vi "PC Streaming Host with slow.vi"() -> ()   [LabVIEW 2012]
uses:
  <vilib>/userdefined/High Color/nirio_resource_hc.ctl
  <vilib>/FPGAPlugInAG/PXI-7951R/niLvFpga_Open_PXI-7951R.vi
  <vilib>/rvi/interface/common/dynamic/niFpgaDynamicAddResources.vi
  <vilib>/Utility/error.llb/Error Cluster From Error Code.vi
  <vilib>/rvi/errors/niLvFpgaAdjustHostInterfaceError.vi
  <vilib>/FPGAPlugInAG/Dynamic/niLvFpga_Close_Dynamic.vi
  <vilib>/rvi/interface/nirviOpenFPGA/nirviOpenFPGA.xnode
  FPGA Bitfiles/ModuDAQ_FPGATarget_TopLevelFPGAw8ra_+uETqx0Rcow.lvbitx
  <vilib>/rvi/interface/nirviReadWriteControl/nirviReadWriteControl.xnode
  <vilib>/rvi/interface/nirviMethod/nirviMethod.xnode
  <vilib>/rvi/interface/nirviCloseFPGA/nirviCloseFPGA.xnode
  <vilib>/ptbypt/NI_PtbyPt.lvlib
  <vilib>/rvi/interface/Simulation/niFpgaSimulationCallBeginRW.vi
  RT_binary.vi
  NiFpgaLv.dll
  <vilib>/FPGAPlugInAG/Dynamic/niLvFpga_ReadFifo_Dynamic.vi
  <vilib>/rvi/errors/niLvFpgaMergeErrorWithErrorCode.vi
panel:
  out "created path":path
  out "File name":string
  out "Total Data Chunks to Write":dbl
  in  "Tab Control":T1(tab)
  in  "Write mode":bool
  out "directory exists - please wait":u8(slide)
  out "directory ok":bool
  in  "Write Enable":bool
  in  "File Path":path=path "D:/Users/reuterc/Desktop"
  out "File Writing Progress (%)":dbl(slide) scale=0.0..100.0
  in  "Slow Control On":bool
  in  "Fast Data On":bool
  in  "Number of Files to Write":u32=1
  in  "IP Address of NIST Time Server":string(combo)
  in  "VISA resource name":refnum<visa-resource-name>="COM5"
  in  "General Cluster":cluster{"Location":i16} {"Location" items=["Purdue", "NIKHEF", "Zurich", "???"]}
  in  "PXI address":T2 caption="RIO Device"
  in  "Channel Cluster":T3={"det_type"=[], "voltage"=[], "Serial numbers"=[], "Sources"=[], "Trigger level"=[4000, 4000, 4000, 4000, 4000, 4000, 4000, 4000], "Channel On/Off"=[], "Number of Channels"=8}
  in  "Testpulse Cluster":T4={"Master Pulser On/Off"=FALSE, "Testpulse Turnaround Time (samples)"=14, "Pulse Separation (samples)"=0, "Pulse duration (samples)"=0}
  out "Samples per Data Chunk":u32
  in  "DAQ Info Cluster":T5={"Data Chunks per File"=1000, "Samples per Waveform"=95, "Pretrigger Samples"=15, "circular buffer length (samples)"=1000, "Waveforms per Data Chunk"=5000} {"Waveforms per Data Chunk" format="%.2p"}
  out "Average Throughput":dbl(graph)
  out "Loop Time":u32
  out "Inst. Throughput":dbl format="%#_6p"
  out "Elements in FIFO":u32(graph)
  out "FIFO Overflow":bool
  out "Current Chunk":u32
  out "Current File":i32
  out "Waveform Graph":dynamicdata(graph)
  out "Channel number displayed":i16=-1
  in  "Arduino read rate (Hz)":dbl=1.0
  out "read buffer":string
  out "array 2":string[](array[string])
  out "Arduino read failed":bool
  out "Slow time":u64
  out "data":dbl[](array[numeric])
  in  "XON Character":u8=17 format="%.0x"
  in  "XOFF Character":u8=19 format="%.0x"
  out "Slow Cluster":T6={"Number of Slow Parameters"=0, "UTC format?"=TRUE, "Sensor Upper bounds"=[85, 1000000, 8000, 8000, 8000, 14000, 99, 33000], "Sensor Lower bounds"=[-40, 0, -8000, -8000, -8000, -14000, 0, -33000], "datanames"=[], "Descriptions"=[]}
  out "FPGA Timestamp (s)":u64
  out "Temperature":dbl(graph)
  out "Pressure":dbl(graph)
  out "magnetic field y coordinate":dbl(graph)
  out "total magnetic field":dbl(graph)
  out "magnetic field z coordinate":dbl(graph)
  out "magnetic field x coordinate":dbl(graph)
  out "humidity":dbl(graph)
  out "XML String":string
  out "Slow XML":string
  out "error out":errorcluster
  out "NIST Time":u64
  out "NIST Time Failed to Read":bool
  in  "Minutes to wait":u32=5 min=3
  out "UTC format":bool=TRUE
  out "Stopped":bool
  in  "stop 2":bool
  in  "stop":bool
  # "Write continuously"
  # "Write finite number of files"
  # "Program will stop when number of Files to Write is Complete OR if stop is pressed."
  # "TODO: Make this look like the \"detectors\" tab"
  # "Waveform/Data Chunk information"
  # "To compare directly on a scope: Horizontal scale: 200 ns/div Vertical scale: ~100 mV/div If 15 pretriggers, delay = 700 ns"
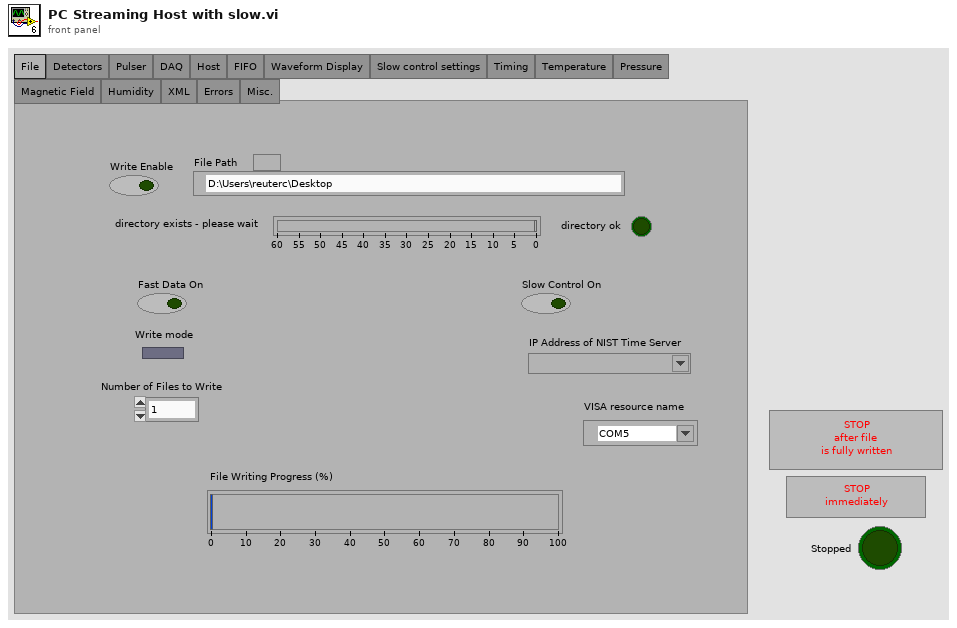
[diagram p1: front panel]
types:
  T1 = enum32{"File", "Detectors", "Pulser", "DAQ", "Host", "FIFO", "Waveform Display", "Slow control settings", "Timing", "Temperature", "Pressure", "Magnetic Field", "Humidity", "XML", "Errors", "Misc."}
  T2 = typedef "nirio_resource_hc.ctl" = tag
  T3 = cluster{"det_type":string[], "voltage":string[], "Serial numbers":string[], "Sources":string[], "Trigger level":i16[], "Channel On/Off":bool[], "Number of Channels":u8}
  T4 = cluster{"Master Pulser On/Off":bool, "Testpulse Turnaround Time (samples)":u32, "Pulse Separation (samples)":u32, "Pulse duration (samples)":u32}
  T5 = cluster{"Data Chunks per File":u32, "Samples per Waveform":u32, "Pretrigger Samples":u32, "circular buffer length (samples)":u32, "Waveforms per Data Chunk":u32}
  T6 = cluster{"Number of Slow Parameters":i32, "UTC format?":bool, "Sensor Upper bounds":i32[], "Sensor Lower bounds":i32[], "datanames":string[], "Descriptions":string[]}
  T7 = enum16{"open", "replace", "create", "open or create", "replace or create", "replace or create with confirmation"}
  T8 = enum16{"big-endian, network order", "native, host order", "little-endian"}
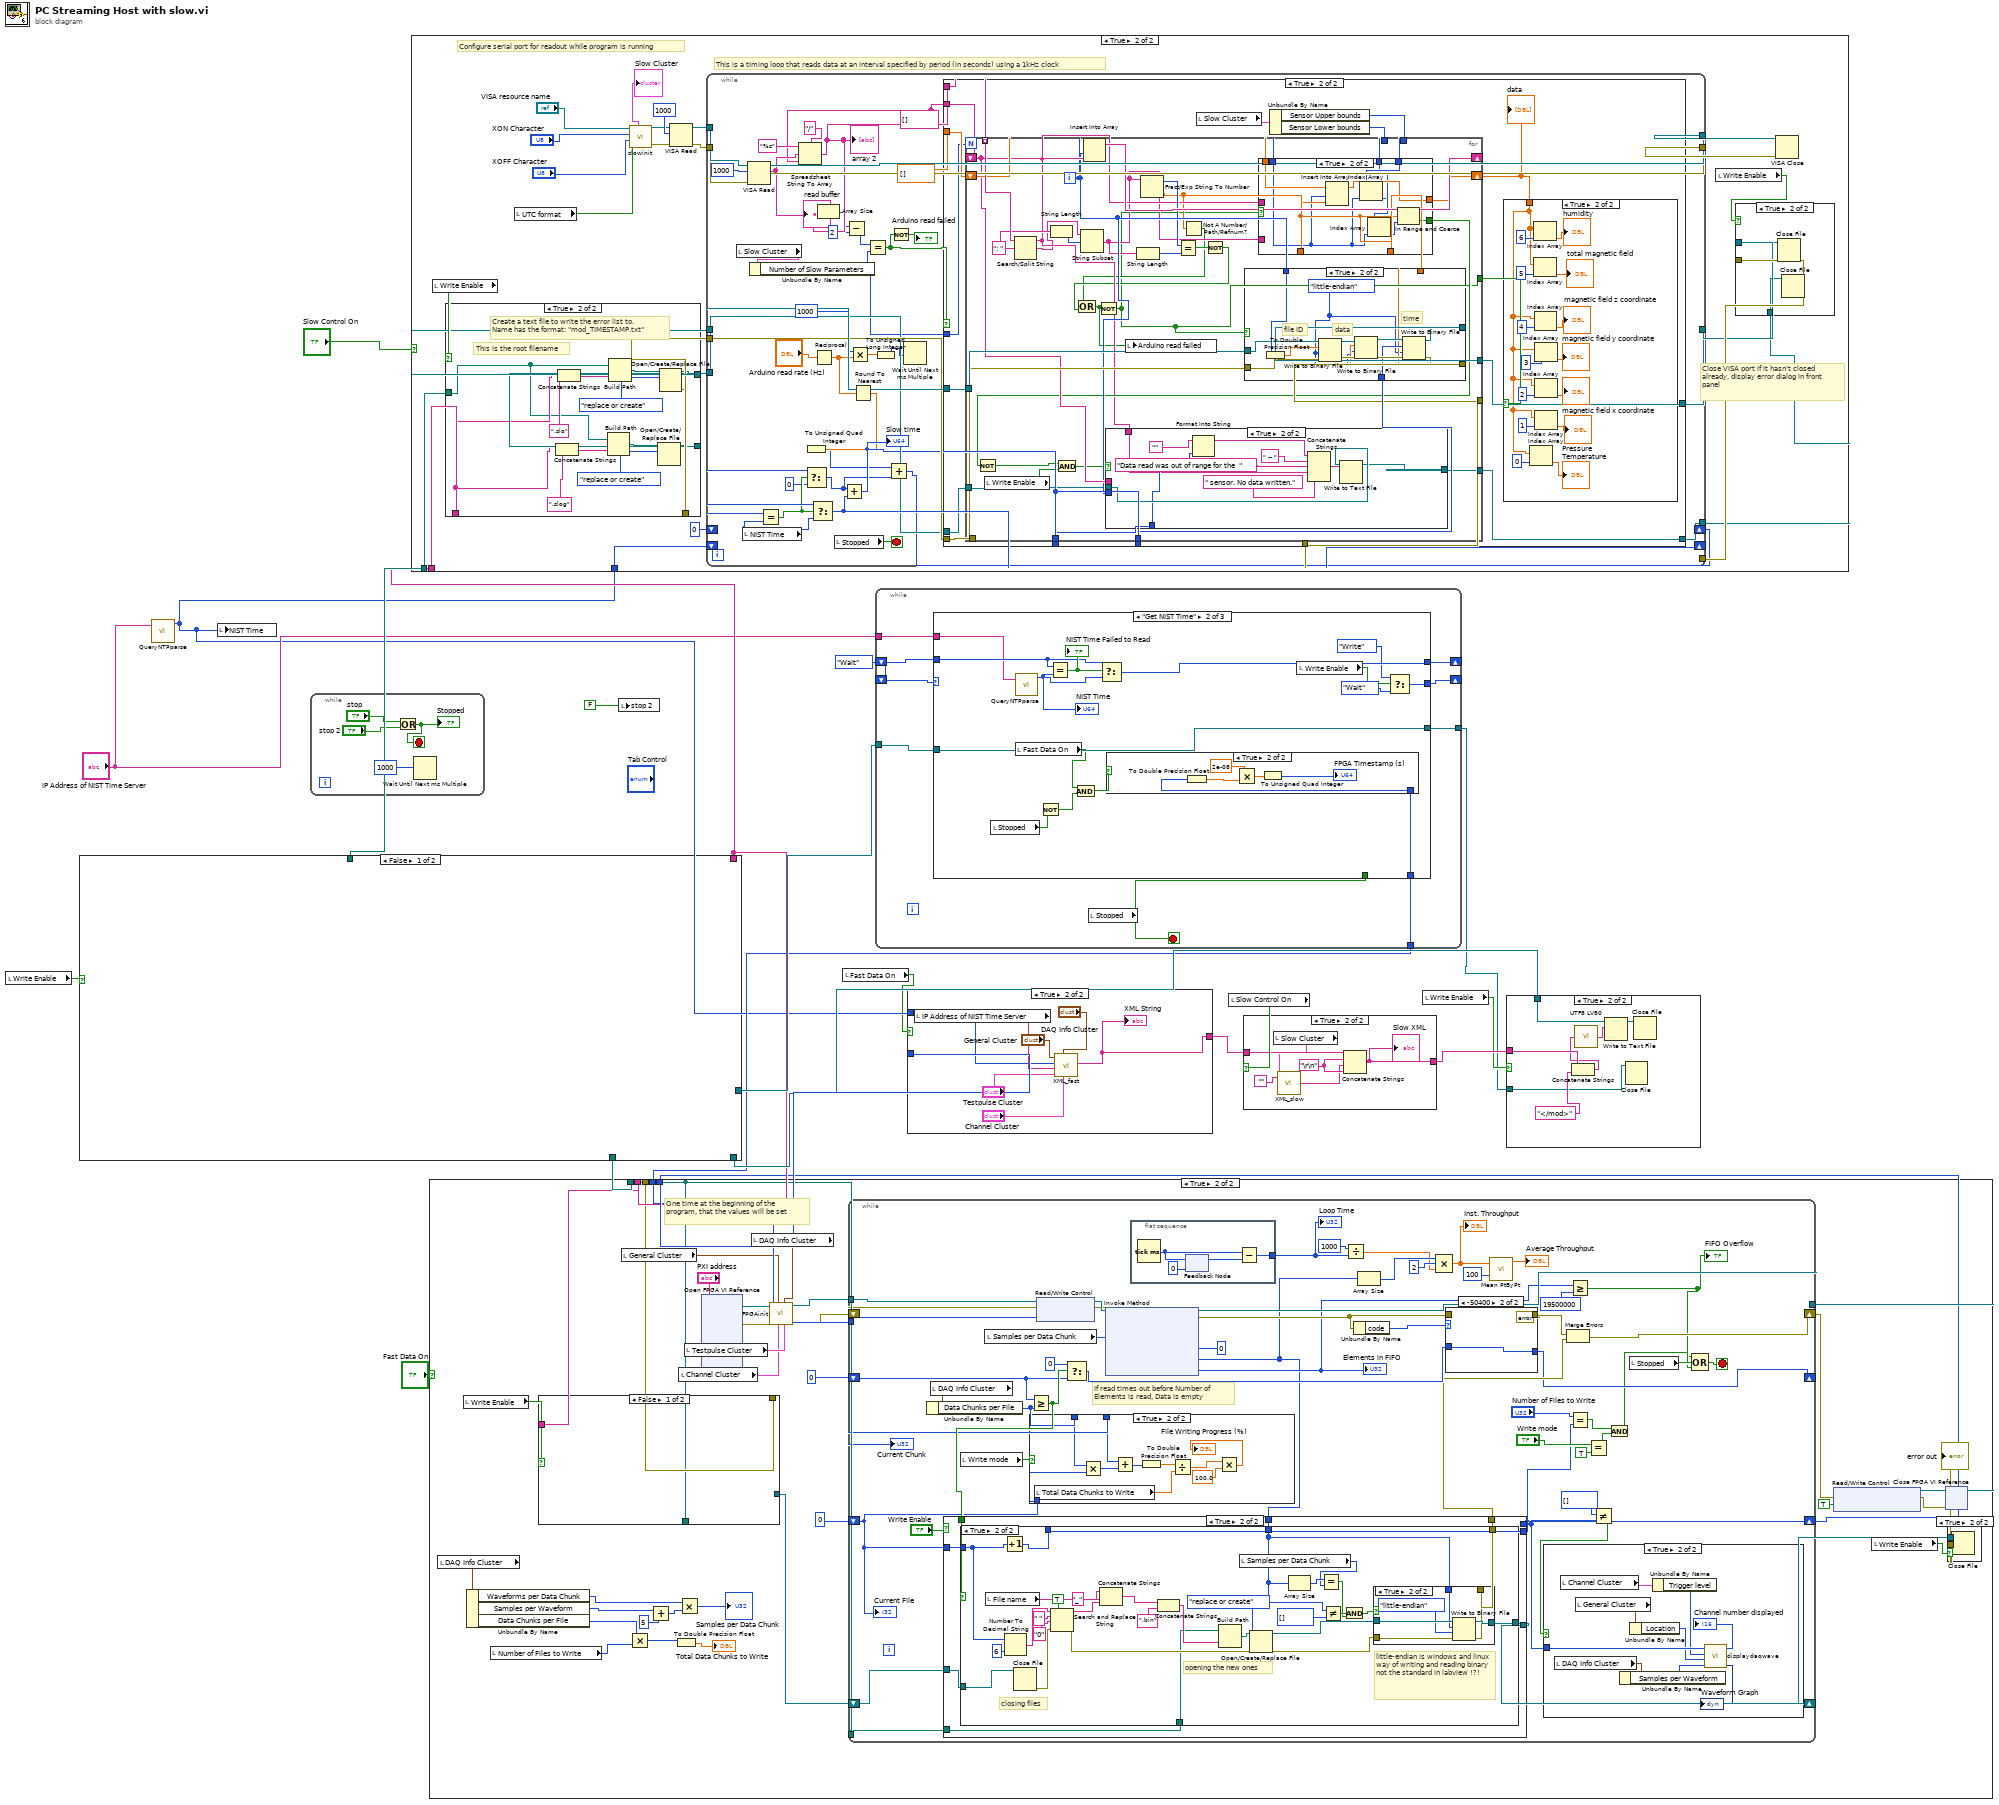
[diagram p0: block diagram]
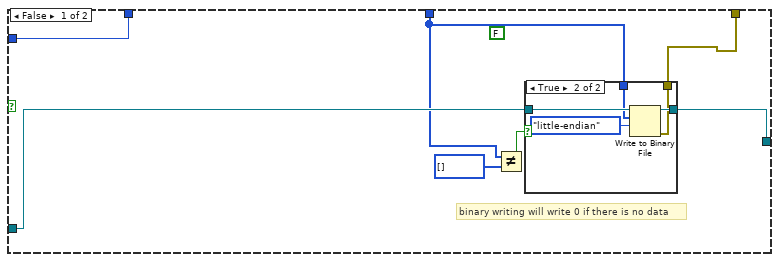
[diagram p10: hidden frame]
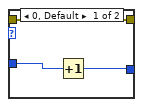
[diagram p13: hidden frame]
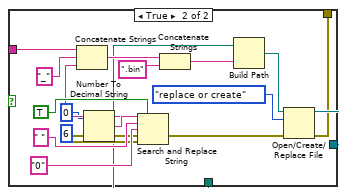
[diagram p14: hidden frame]
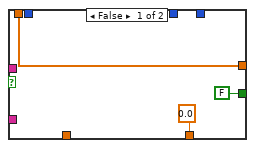
[diagram p18: hidden frame]
diagram:
  n1 = local read "Write Enable"() -> (w17:bool)
  n2 = case shown="False" w17 {
    tunnel: [_ w37] -> w18
    tunnel: [_ w32] -> w14
    tunnel: [_ w24] -> w12
    tunnel: [_ w22] -> w11
    tunnel: [_ w21] -> w9
    frame False {
    }
    frame True {
      # "additional folder"
      n3 = while {
        tunnel: [w50] -> w34
        tunnel: [w41] -> w35
        tunnel: [w41] -> w32
        tunnel: [w40] -> w22
        stop <- w47 stop-if-true
        w42 = "\\" ("string")
        w53 = TRUE ("UTC format")
        # "modulation experiment"
        # "purdue"
        # "timestamp for the file name and the folder"
        n4 = Get Date/Time In Seconds() -> (seconds since 1Jan1904=w54:timestamp)
        n5 = Format Date/Time String(time format string (%c)="%Y%m%d_%H%M", seconds (now)=w54, UTC format=w53) -> (date/time string=w43:string)
        n6 = Concatenate Strings("mx" ("string"), "_" ("string"), "p_" ("string"), w43) -> (w40:string)
        "File name" <- w40
        n7 = Path To String(path="File Path") -> (string=w56:string)
        n8 = Concatenate Strings(w56, w42, w40, w42) -> (w57:string)
        n9 = String To Path(string=w57) -> (path=w51:path)
        n10 = call <vilib>:"Check if File or Folder Exists.vi"("path"=w51) -> ("error out"=w50:errorcluster, "file or folder exists?"=w49:bool, "dup path"=w41:path)  [unwired: 8 in]
        "created path" <- w41
        n11 = case shown="True" w49 {
          frame False {
          }
          frame True {
            n12 = Format Date/Time String(time format string (%c)="%S") -> (date/time string=w61:string)  [unwired: 2 in]
            n13 = Decimal String To Number(string=w61) -> (number=w59:i32)  [unwired: 2 in, 1 out]
            n14 = Subtract(x=60, y=w59) -> (x-y=→"directory exists - please wait":i32)
          }
        }
        n15 = Not(x=w49) -> (.not. x?=w47:bool)
        "directory ok" <- w47
        n16 = Wait (ms)(milliseconds to wait=1000) -> ()  [unwired: 1 out]
        "UTC format" <- w53
      }
      n17 = Create Folder(path (use dialog)=w35, error in=w34) -> (created path=w21:path)  [unwired: 1 in, 2 out]
      n18 = Concatenate Strings(w22, ".tim" ("string")) -> (w36:string)
      n19 = Build Path(base path=w21, name or relative path=w36) -> (appended path=w33:path)
      n20 = Concatenate Strings(w22, ".XML" ("substring (\"\")")) -> (w28:string)
      n21 = Open/Create/Replace File(file path (use dialog)=w33, operation (0:open)=T7."replace or create") -> (refnum out=w37:refnum<file>)  [unwired: 4 in, 2 out]
      n22 = Build Path(base path=w21, name or relative path=w28) -> (appended path=w27:path)
      n23 = call "UTF8 LV80.vi"("text"="<mod>") -> ("utf-8 text out"=w31:string)
      n24 = Open/Create/Replace File(file path (use dialog)=w27, operation (0:open)=T7."replace or create") -> (refnum out=w30:refnum<file>, error out=w29:errorcluster)  [unwired: 4 in, 1 out]
      n25 = Write to Text File(file (use dialog)=w30, text=w31, error in=w29) -> (refnum out=w24:refnum<file>)  [unwired: 1 in, 2 out]
    }
  }
  n26 = call "QueryNTPparse.vi"("IP Address of NIST Server"="IP Address of NIST Time Server") -> ("NTP Time"=w7:u64)  [unwired: 1 in, 2 out]
  n27 = local write "NIST Time"(w7) -> ()
  n28 = while {
    stop <- w63 stop-if-true
    n29 = Or(x="stop", y="stop 2") -> (x .or. y?=w63:bool)
    "Stopped" <- w63
    n30 = Wait Until Next ms Multiple(millisecond multiple=u32 1000 ("y")) -> ()  [unwired: 1 out]
  }
  n31 = case shown="True" "Slow Control On" {
    tunnel: w14 -> [_ w82]
    tunnel: w7 -> [_ w80]
    tunnel: w11 -> [_ w79]
    frame False {
    }
    frame True {
      # "This is a timing loop that reads data at an interval specified by period (in seconds) using a 1kHz clock"
      # "Configure serial port for readout while program is running"
      # "Close VISA port if it hasn't closed already, display error dialog in front panel"
      n32 = local read "Write Enable"() -> (w89:bool)
      n33 = case shown="True" w89 {
        tunnel: [_ w252] -> w86
        tunnel: [_ w249] -> w84
        tunnel: w82 -> [_ w242]
        tunnel: w79 -> [_ w244]
        tunnel: [_ w243] -> w75
        frame False {
        }
        frame True {
          # "This is the root filename"
          # "Create a text file to write the error list to.  \nName has the format: \"mod_TIMESTAMP.txt\""
          n34 = Concatenate Strings(w244, ".slog") -> (w245:string)
          n35 = Concatenate Strings(w244, ".slo") -> (w250:string)
          n36 = Build Path(base path=w242, name or relative path=w245) -> (appended path=w246:path)
          n37 = Build Path(base path=w242, name or relative path=w250) -> (appended path=w251:path)
          n38 = Open/Create/Replace File(file path (use dialog)=w246, operation (0:open)=T7."replace or create") -> (refnum out=w243:refnum<file>)  [unwired: 4 in, 2 out]
          n39 = Open/Create/Replace File(file path (use dialog)=w251, operation (0:open)=T7."replace or create") -> (refnum out=w252:refnum<file>, error out=w249:errorcluster)  [unwired: 4 in, 1 out]
        }
      }
      n40 = local read "UTC format"() -> (w70:bool)
      n41 = call "slowinit.vi"("UTC format"=w70, "XOFF Character"="XOFF Character", "XON Character"="XON Character", "VISA resource name"="VISA resource name") -> ("error IO"=w68:errorcluster, "VISA resource name out"=w69:refnum<visa-resource-name>, "Slow Cluster"=→"Slow Cluster":T6)  [unwired: 5 in]
      n42 = VISA Read(VISA resource name=w69, byte count=u32 1000, error in (no error)=w68) -> (VISA resource name out=w78:refnum<visa-resource-name>, error out=w77:errorcluster)  [unwired: 2 out]
      n43 = while {
        tunnel: w78 -> [w130]
        tunnel: w77 -> [w129]
        tunnel: [w128] -> w88
        tunnel: [w127] -> w87
        shift-right: [w117] -> _
        shift-left: w80 -> [w121]
        shift-right: [w102] -> _
        shift-left: 0 -> [w119]
        tunnel: w84 -> [w115]
        tunnel: [w114] -> w83
        tunnel: w86 -> [w123]
        tunnel: [w113] -> w81
        tunnel: w75 -> [w110]
        tunnel: [w108] -> w74
        stop <- w116 stop-if-true
        w107 = string[] [] ("array type (2D Dbl)")
        n44 = local read "Slow Cluster"() -> (w95:T6)
        n45 = local read "NIST Time"() -> (w122:u64)
        n46 = VISA Read(VISA resource name=w130, byte count=u32 1000, error in (no error)=w129) -> (VISA resource name out=w128:refnum<visa-resource-name>, read buffer=w126:string, error out=w127:errorcluster)  [unwired: 1 out]
        "read buffer" <- w126
        n47 = Unbundle By Name(w95) -> ("Number of Slow Parameters"=w94:i32)
        n48 = Equal?(x=w121, y=w122) -> (x = y?=w120:bool)
        n49 = Spreadsheet String To Array(delimiter (Tab)="/", format string="%s", spreadsheet string=w126, array type (2D Dbl)=w107) -> (array=w96:string[])
        "array 2" <- w96
        n50 = Select(t=w119, s=w120, f=0) -> (s? t:f=w103:u64)
        n51 = Select(t=w121, s=w120, f=w122) -> (s? t:f=w117:u64)
        n52 = Reciprocal(x="Arduino read rate (Hz)") -> (1/x=w99:dbl)
        n53 = Array Size(array=w96) -> (size(s)=w93:i32)
        n54 = local read "Stopped"() -> (w116:bool)
        n55 = Add(x=w103, y=w117) -> (x+y=w109:u64)
        "Slow time" <- w109
        n56 = Subtract(x=w93, y=2) -> (x-y=w91:i32)
        n57 = Multiply(x=u32 1000 ("millisecond multiple"), y=w99) -> (x*y=w101:dbl)
        n58 = Round To Nearest(number=w99) -> (nearest integer value=w98:dbl)
        n59 = To Unsigned Quad Integer(1:w98) -> (0:w97:u64)
        n60 = Equal?(x=w91, y=w94) -> (x = y?=w112:bool)
        n61 = To Unsigned Long Integer(number=w101) -> (unsigned 32bit integer=w100:u32)
        n62 = Add(x=w97, y=w103) -> (x+y=w102:u64)
        n63 = Not(x=w112) -> (.not. x?=→"Arduino read failed":bool)
        n64 = Wait Until Next ms Multiple(millisecond multiple=w100) -> ()  [unwired: 1 out]
        n65 = case shown="True" w112 {
          tunnel: w96 -> [_ w151]
          tunnel: w107 -> [_ w150]
          tunnel: w123 -> [w133 w149]
          tunnel: w109 -> [_ w148]
          tunnel: w115 -> [w134 w147]
          tunnel: [w134 w146] -> w114
          tunnel: [w133 w145] -> w113
          tunnel: w110 -> [w132 w143]
          tunnel: w109 -> [_ w142]
          tunnel: [w132 w141] -> w108
          tunnel: dbl[] [] ("array type (2D Dbl)") -> [_ w139]
          tunnel: w94 -> [_ w135]
          frame False {
          }
          frame True {
            n66 = local read "Slow Cluster"() -> (w138:T6)
            n67 = Unbundle By Name(w138) -> ("Sensor Upper bounds"=w137:i32[], "Sensor Lower bounds"=w136:i32[])
            n68 = for {
              N: w135 -> [_]
              tunnel: w151 -> [w200] mode=indexing
              shift-right: [w199] -> _
              shift-left: w150 -> [w190]
              shift-right: [w197] -> w144
              shift-left: w139 -> [w198]
              tunnel: w149 -> [w196]
              tunnel: [w195] -> w145
              tunnel: w148 -> [w194]
              tunnel: w147 -> [w193]
              tunnel: [w192] -> w146
              tunnel: w143 -> [w188]
              tunnel: w142 -> [w187]
              tunnel: [w186] -> w141
              tunnel: [w169] -> w140
              tunnel: w137 -> [w168]
              tunnel: w136 -> [w167]
              i -> [w189]
              w179 = ": " ("search string/char (-)")
              n69 = local read "Write Enable"() -> (w180:bool)
              n70 = Search/Split String(string=w200, search string/char (-)=w179) -> (substring before match=w177:string, match + rest of string=w175:string)  [unwired: 1 in, 1 out]
              n71 = String Length(string=w179) -> (length=w178:i32)
              n72 = String Subset(string=w175, offset (0)=w178) -> (substring=w176:string)  [unwired: 1 in]
              n73 = Insert Into Array(array=w190, index=w189, new element=w177) -> (w199:string[])
              n74 = String Length(string=w176) -> (length=w183:i32)
              n75 = Fract/Exp String To Number(string=w176) -> (offset past number=w184:i32, number=w172:dbl)  [unwired: 3 in]
              n76 = Equal?(x=w184, y=w183) -> (x = y?=w182:bool)
              n77 = Not A Number/Path/Refnum?(number/path/refnum=w172) -> (NaN/Path/Refnum?=w171:bool)
              n78 = Not(x=w182) -> (.not. x?=w173:bool)
              n79 = Compound Arithmetic op=OR(w171, w173) -> (w174:bool)
              n80 = Not(x=w174) -> (.not. x?=w169:bool)
              n81 = local write "Arduino read failed"(w174) -> ()
              n82 = case shown="True" w169 {
                tunnel: w198 -> [w201 w212]
                tunnel: [w201 w210] -> w197
                tunnel: w177 -> [_ _]
                tunnel: [0.0 w209] -> w191
                tunnel: w189 -> [_ w208]
                tunnel: [FALSE w211] -> w185
                tunnel: w176 -> [_ _]
                tunnel: w172 -> [_ w209]
                tunnel: w168 -> [_ w207]
                tunnel: w167 -> [_ w206]
                frame False {
                }
                frame True {
                  n83 = Insert Into Array(array=w212, index=w208, new element=w209) -> (w210:dbl[])
                  n84 = Index Array(array=w207, index=w208) -> (element=w205:i32)
                  n85 = Index Array(array=w206, index=w208) -> (element=w204:i32)
                  n86 = In Range and Coerce(upper limit=w205, x=w209, lower limit=w204) -> (In Range?=w211:bool)  [unwired: 1 out]
                }
              }
              n87 = Not(x=w185) -> (.not. x?=w181:bool)
              n88 = And(x=w181, y=w180) -> (x .and. y?=w170:bool)
              n89 = case shown="True" w170 {
                tunnel: w190 -> [_ _]
                tunnel: w189 -> [_ _]
                tunnel: w188 -> [w213 w221]
                tunnel: w187 -> [_ w219]
                tunnel: [w213 w217] -> w186
                tunnel: w177 -> [_ w214]
                frame False {
                }
                frame True {
                  n90 = Format Into String(initial string="", w219) -> (resulting string=w218:string)  [unwired: 2 in, 1 out]
                  n91 = Concatenate Strings(w218, " -- " ("format string"), "Data read was out of range for the  " ("format string"), w214, " sensor. No data written." ("format string")) -> (w215:string)
                  n92 = Write to Text File(file (use dialog)=w221, text=w215) -> (refnum out=w217:refnum<file>)  [unwired: 2 in, 2 out]
                }
              }
              n93 = case shown="True" w169 {
                tunnel: [w225 w232] -> w195
                tunnel: w196 -> [w225 w235]
                tunnel: w189 -> [_ w236]
                tunnel: w194 -> [_ w229]
                tunnel: w193 -> [w224 w238]
                tunnel: [w224 w230] -> w192
                tunnel: w191 -> [_ w228]
                frame False {
                }
                frame True {
                  w226 = T8."little-endian" ("byte order (0:big-endian, network order)")
                  # "time"
                  # "data"
                  # "file ID"
                  n94 = To Double Precision Float(number=w236) -> (double precision float=w227:dbl)
                  n95 = Write to Binary File(file (use dialog)=w235, data=w227, error in=w238, 9:w226) -> (refnum out=w234:refnum<file>, error out=w237:errorcluster)  [unwired: 2 in, 1 out]
                  n96 = Write to Binary File(file (use dialog)=w234, data=w228, error in=w237, 9:w226) -> (refnum out=w233:refnum<file>, error out=w231:errorcluster)  [unwired: 2 in, 1 out]
                  n97 = Write to Binary File(file (use dialog)=w233, data=w229, error in=w231, 9:w226) -> (refnum out=w232:refnum<file>, error out=w230:errorcluster)  [unwired: 2 in, 1 out]
                }
              }
            }
            "data" <- w144
            n98 = case shown="True" w140 {
              tunnel: w144 -> [_ w159]
              frame False {
              }
              frame True {
                n99 = Index Array(array=w159, index=0) -> (element=→"Temperature":dbl)
                n100 = Index Array(array=w159, index=6) -> (element=→"humidity":dbl)
                n101 = Index Array(array=w159, index=5) -> (element=→"total magnetic field":dbl)
                n102 = Index Array(array=w159, index=4) -> (element=→"magnetic field z coordinate":dbl)
                n103 = Index Array(array=w159, index=3) -> (element=→"magnetic field y coordinate":dbl)
                n104 = Index Array(array=w159, index=2) -> (element=→"magnetic field x coordinate":dbl)
                n105 = Index Array(array=w159, index=1) -> (element=→"Pressure":dbl)
              }
            }
          }
        }
      }
      n106 = local read "Write Enable"() -> (w90:bool)
      n107 = case shown="True" w90 {
        tunnel: w81 -> [_ w241]
        tunnel: w83 -> [_ w240]
        tunnel: w74 -> [_ w239]
        frame False {
        }
        frame True {
          n108 = Close File(refnum=w241, error in=w240) -> ()  [unwired: 2 out]
          n109 = Close File(refnum=w239) -> ()  [unwired: 1 in, 2 out]
        }
      }
      n110 = VISA Close(VISA resource name=w88, error in (no error)=w87) -> ()  [unwired: 1 out]
    }
  }
  n111 = case shown="True" "Fast Data On" {
    tunnel: [_ w290] -> _
    tunnel: [_ w277] -> w13
    tunnel: w11 -> [_ w276]
    tunnel: w9 -> [_ w275]
    tunnel: [_ w274] -> w8
    frame False {
    }
    frame True {
      # "One time at the beginning of the program, that the values will be set"
      n112 = local read "DAQ Info Cluster"() -> (w272:T5)
      n113 = local read "Write Enable"() -> (w289:bool)
      n114 = Unbundle By Name(w272) -> ("Waveforms per Data Chunk"=w257:u32, "Samples per Waveform"=w258:u32, "Data Chunks per File"=w259:u32)
      n115 = local read "Number of Files to Write"() -> (w260:u32)
      n116 = case shown="False" w289 {
        tunnel: [_ w435] -> w290
        tunnel: [_ w443] -> w288
        tunnel: w276 -> [_ w434]
        tunnel: w275 -> [_ w433]
        frame False {
        }
        frame True {
          n117 = Number To Decimal String(number=0, width (-)=i16 6) -> (decimal integer string=w450:string)
          n118 = Search and Replace String(replace all?=TRUE ("replace all? (F)"), input string=w450, search string=" ", replace string="0" ("replace string (\"\")")) -> (result string=w440:string, error out=w445:errorcluster)  [unwired: 4 in, 2 out]
          n119 = Concatenate Strings(w434, "_" ("string"), w440) -> (w438:string)
          n120 = Concatenate Strings(w438, ".bin" ("substring (\"\")")) -> (w442:string)
          n121 = Build Path(base path=w433, name or relative path=w442) -> (appended path=w446:path)
          n122 = Open/Create/Replace File(file path (use dialog)=w446, error in=w445, operation (0:open)=T7."replace or create") -> (refnum out=w443:refnum<file>, error out=w435:errorcluster)  [unwired: 3 in, 1 out]
        }
      }
      n123 = local read "General Cluster"() -> (w266:cluster{"Location":i16})
      n124 = Multiply(x=w259, y=w260) -> (x*y=w264:u32)
      n125 = Add(x=w258, y=u32 5) -> (x+y=w262:u32)
      n126 = To Double Precision Float(number=w264) -> (double precision float=→"Total Data Chunks to Write":dbl)
      n127 = Multiply(x=w257, y=w262) -> (x*y=→"Samples per Data Chunk":u32)
      n128 = local read "Channel Cluster"() -> (w265:T3)
      n129 = local read "Testpulse Cluster"() -> (w267:T4)
      n130 = xnode "Open FPGA VI Reference"("resource name"="PXI address") -> ("FPGA VI Reference Out"=w271:refnum<k20>, "error out"=w270:errorcluster)  [unwired: 1 in]
      n131 = local read "DAQ Info Cluster"() -> (w255:T5)
      n132 = call "FPGAinit.vi"("Testpulse Cluster"=w267, "DAQ Info Cluster"=w255, "Channel Cluster"=w265, "General Cluster"=w266, "error in"=w270, "FPGA VI Reference In"=w271) -> ("error out"=w268:errorcluster, "FPGA VI Reference Out"=w269:refnum<k20>)  [unwired: 4 in]
      n133 = while {
        shift-right: [w326] -> w280
        shift-left: w268 -> [w314]
        shift-right: [w322] -> _
        shift-left: u32 0 -> [w319]
        shift-right: [w303] -> w277
        shift-left: 0 ("number") -> [w307]
        shift-right: [w323] -> w284
        shift-left: w288 -> [w324]
        tunnel: [w342] -> w281
        tunnel: w275 -> [w315]
        tunnel: [w311] -> w274
        tunnel: w269 -> [w295]
        stop <- w308 stop-if-true
        # "If read times out before Number of Elements is read, Data is empty"
        n134 = local read "DAQ Info Cluster"() -> (w297:T5)
        n135 = Unbundle By Name(w297) -> ("Data Chunks per File"=w296:u32)
        n136 = local read "Write mode"() -> (w316:bool)
        n137 = local read "Samples per Data Chunk"() -> (w294:u32)
        n138 = Greater Or Equal?(x=w319, y=w296) -> (x >= y?=w328:bool)
        n139 = case shown="True" w316 {
          tunnel: w307 -> [_ w361]
          tunnel: w319 -> [_ w359]
          tunnel: w296 -> [_ w352]
          frame False {
          }
          frame True {
            n140 = local read "Total Data Chunks to Write"() -> (w356:dbl)
            n141 = Multiply(x=w352, y=w361) -> (x*y=w360:u32)
            n142 = Add(x=w359, y=w360) -> (x+y=w358:u32)
            n143 = To Double Precision Float(number=w358) -> (double precision float=w357:dbl)
            n144 = Divide(x=w357, y=w356) -> (x/y=w354:dbl)
            n145 = Multiply(x=w354, y=100.0) -> (x*y=→"File Writing Progress (%)":dbl)
          }
        }
        n146 = xnode "Read/Write Control"("FPGA VI Reference In"=w295, "error in"=w314) -> ("FPGA VI Reference Out"=w313:refnum<k20>, "error out"=w312:errorcluster, "Timestamp"=w311:u64)
        n147 = Select(t=u32 0, s=w328, f=w319) -> (s? t:f=w329:u32)
        n148 = xnode "Invoke Method"("FPGA VI Reference In"=w313, "error in"=w312, "Number of Elements"=w294, "Timeout (ms)"=0) -> ("FPGA VI Reference Out"=w342:refnum<k20>, "error out"=w339:errorcluster, "Data"=w317:i16[], "Elements Remaining"=w318:u32)
        "Elements in FIFO" <- w318
        n149 = case shown="True" "Write Enable" {
          tunnel: w317 -> [w367 w372]
          tunnel: [w367 _] -> w300
          tunnel: w328 -> [_ w376]
          tunnel: [_ w375] -> w325
          tunnel: [w368 w374] -> w323
          tunnel: w324 -> [w368 w373]
          tunnel: w315 -> [_ w371]
          tunnel: w307 -> [w366 w370]
          tunnel: [w366 w369] -> w303
          frame False {
          }
          frame True {
            n150 = case shown="True" w376 {
              tunnel: w372 -> [w379 w398]
              tunnel: [w378 w400] -> w375
              tunnel: w373 -> [w383 w413]
              tunnel: [w382 w406] -> w374
              tunnel: w371 -> [_ w393]
              tunnel: w370 -> [w377 w392]
              tunnel: [w377 w391] -> w369
              frame False {
                (unwired) FALSE
                # "binary writing will write 0 if there is no data"
                n151 = Not Equal?(x=w379, y=i16[] []) -> (x != y?=w380:bool)
                n152 = case shown="True" w380 {
                  tunnel: w383 -> [w384 w389]
                  tunnel: [w384 w388] -> w382
                  tunnel: [_ w387] -> w378
                  tunnel: w379 -> [_ w385]
                  frame False {
                  }
                  frame True {
                    n153 = Write to Binary File(file (use dialog)=w389, data=w385, 9:T8."little-endian" ("byte order (0:big-endian, network order)")) -> (refnum out=w388:refnum<file>, error out=w387:errorcluster)  [unwired: 3 in, 1 out]
                  }
                }
              }
              frame True {
                # "opening the new ones"
                # "closing files"
                # "little-endian is windows and linux way of writing and reading binary not the standard in labview !?!"
                n154 = local read "File name"() -> (w394:string)
                n155 = Increment(x=w392) -> (x+1=w391:i32)
                n156 = Number To Decimal String(number=w392, width (-)=i16 6) -> (decimal integer string=w415:string)
                n157 = Close File(refnum=w413) -> (error out=w412:errorcluster)  [unwired: 1 in, 1 out]
                n158 = Search and Replace String(replace all?=TRUE ("replace all? (F)"), input string=w415, search string=" ", replace string="0" ("replace string (\"\")"), error in=w412) -> (result string=w405:string, error out=w411:errorcluster)  [unwired: 3 in, 2 out]
                n159 = Concatenate Strings(w394, "_" ("string"), w405) -> (w401:string)
                n160 = Concatenate Strings(w401, ".bin" ("substring (\"\")")) -> (w403:string)
                n161 = Build Path(base path=w393, name or relative path=w403) -> (appended path=w410:path)
                n162 = local read "Samples per Data Chunk"() -> (w390:u32)
                n163 = Open/Create/Replace File(file path (use dialog)=w410, error in=w411, operation (0:open)=T7."replace or create") -> (refnum out=w407:refnum<file>, error out=w408:errorcluster)  [unwired: 3 in, 1 out]
                n164 = Array Size(array=w398) -> (size(s)=w397:i32)
                n165 = Equal?(x=w397, y=w390) -> (x = y?=w396:bool)
                n166 = Not Equal?(x=w398, y=i16[] []) -> (x != y?=w399:bool)
                n167 = And(x=w399, y=w396) -> (x .and. y?=w395:bool)
                n168 = case shown="True" w395 {
                  tunnel: w408 -> [w420 w427]
                  tunnel: w407 -> [w421 w426]
                  tunnel: [w421 w425] -> w406
                  tunnel: [w420 w424] -> w400
                  tunnel: w398 -> [_ w423]
                  frame False {
                  }
                  frame True {
                    n169 = Write to Binary File(file (use dialog)=w426, data=w423, error in=w427, 9:T8."little-endian" ("byte order (0:big-endian, network order)")) -> (refnum out=w425:refnum<file>, error out=w424:errorcluster)  [unwired: 2 in, 1 out]
                  }
                }
              }
            }
          }
        }
        n170 = flat-sequence {
          tunnel: [w365] -> w333
          frame #0 {
            n171 = Tick Count (ms)() -> (millisecond timer value=w364:u32)
            n172 = feedback #1(u32 0 ("millisecond timer value")) -> (w363:u32)
            n173 = feedback-in #1(w364) -> ()
            n174 = Subtract(x=w364, y=w363) -> (x-y=w365:u32)
          }
        }
        n175 = Divide(x=u32 1000, y=w333) -> (x/y=w335:dbl)
        n176 = Unbundle By Name(w339) -> ("code"=w340:i32)
        n177 = Array Size(array=w317) -> (size(s)=w338:i32)
        n178 = Compound Arithmetic op=MULTIPLY(w338, 2 ("y"), w335) -> (w332:dbl)
        "Inst. Throughput" <- w332
        n179 = case shown="-50400" w340 {
          tunnel: [w430 errorcluster {"status"=FALSE, "code"=0, "source"=""} ("error constant")] -> w327
          tunnel: w339 -> [w430 _]
          tunnel: w329 -> [w429 w431]
          tunnel: [w428 w431] -> w322
          frame 0, Default {
            n180 = Increment(x=w429) -> (x+1=w428:u32)
          }
          frame -50400 {
          }
        }
        n181 = call <vilib>:"Mean PtByPt.vi"("x"=w332, "sample length"=100) -> ("mean"=→"Average Throughput":dbl)  [unwired: 2 in, 1 out]
        n182 = Merge Errors(w327, w325) -> (w326:errorcluster)
        n183 = Greater Or Equal?(x=w318, y=u32 19500000) -> (x >= y?=w309:bool)
        "FIFO Overflow" <- w309
        n184 = Equal?(x="Number of Files to Write", y=w303) -> (x = y?=w302:bool)
        n185 = Equal?(x="Write mode", y=TRUE) -> (x = y?=w301:bool)
        n186 = Not Equal?(x=i16[] [], y=w300) -> (x != y?=w298:bool)
        n187 = case shown="True" w298 {
          tunnel: w300 -> [_ w351]
          frame False {
          }
          frame True {
            n188 = local read "DAQ Info Cluster"() -> (w345:T5)
            n189 = local read "Channel Cluster"() -> (w349:T3)
            n190 = local read "General Cluster"() -> (w347:cluster{"Location":i16})
            n191 = Unbundle By Name(w345) -> ("Samples per Waveform"=w344:u32)
            n192 = Unbundle By Name(w347) -> ("Location"=w346:i16)
            n193 = Unbundle By Name(w349) -> ("Trigger level"=w348:i16[])
            n194 = call "displaydaqwave.vi"("Samples per Waveform"=w344, "Location"=w346, "Trigger level"=w348, "Waveform from DAQ"=w351) -> ("Waveform Graph"=→"Waveform Graph":dynamicdata, "Channel number displayed"=→"Channel number displayed":i16)  [unwired: 6 in]
          }
        }
        n195 = And(x=w302, y=w301) -> (x .and. y?=w293:bool)
        n196 = local read "Stopped"() -> (w310:bool)
        n197 = Compound Arithmetic op=OR(w293, w310, w309) -> (w308:bool)
        "Loop Time" <- w333
        "Current Chunk" <- w319
        "Current File" <- w307
      }
      n198 = xnode "Read/Write Control"("FPGA VI Reference In"=w281, "error in"=w280, "Stop FPGA and exit"=TRUE) -> ("FPGA VI Reference Out"=w273:refnum<k20>, "error out"=w283:errorcluster)
      n199 = local read "Write Enable"() -> (w286:bool)
      n200 = xnode "Close FPGA VI Reference"("FPGA VI Reference In"=w273, "error in"=w283) -> ("error out"=w287:errorcluster)
      "error out" <- w287
      n201 = case shown="True" w286 {
        tunnel: w287 -> [_ w291]
        tunnel: w284 -> [_ w292]
        frame False {
        }
        frame True {
          n202 = Close File(refnum=w292, error in=w291) -> ()  [unwired: 2 out]
        }
      }
    }
  }
  n203 = local write "stop 2"(FALSE ("stop 2")) -> ()
  n204 = local read "Fast Data On"() -> (w6:bool)
  n205 = while {
    shift-right: [w458] -> _
    shift-left: enum16{"Wait", "Get NIST Time", "Write"}."Wait" -> [w459]
    shift-right: [w457] -> _
    shift-left: _ -> [w456]
    tunnel: w18 -> [w455]
    tunnel: [w454] -> w1
    tunnel: "IP Address of NIST Time Server" -> [w453]
    tunnel: w8 -> [w451]
    stop <- w452 stop-if-true
    n206 = local read "Stopped"() -> (w452:bool)
    n207 = case shown="\"Get NIST Time\"" w459 {
      tunnel: [w464 w480 enum16{"Wait", "Get NIST Time", "Write"}."Wait"] -> w458
      tunnel: [w463 w488 w498] -> w457
      tunnel: w456 -> [w463 w485 w498]
      tunnel: w455 -> [w462 w484 w504]
      tunnel: [w462 w484 w503] -> w454
      tunnel: w452 -> [w461 _ _]
      tunnel: w453 -> [_ w479 _]
      tunnel: w451 -> [_ w474 _]
      frame "Wait", Default {
        n208 = while {
          tunnel: [enum16{"Wait", "Get NIST Time", "Write"}."Get NIST Time"] -> w464
          tunnel: w461 -> [_]
          tunnel: "Minutes to wait" -> [w466]
          i -> [w469]
          stop <- w470 stop-if-true
          n209 = Multiply(x=60, y=w466) -> (x*y=w465:u32)
          n210 = Greater Or Equal?(x=w469, y=w465) -> (x >= y?=w471:bool)
          n211 = local read "Stopped"() -> (w468:bool)
          n212 = Or(x=w471, y=w468) -> (x .or. y?=w470:bool)
          n213 = Wait Until Next ms Multiple(millisecond multiple=u32 1000 ("y")) -> ()  [unwired: 1 out]
        }
      }
      frame "Get NIST Time" {
        n214 = local read "Stopped"() -> (w475:bool)
        n215 = call "QueryNTPparse.vi"("IP Address of NIST Server"=w479) -> ("NTP Time"=w487:u64)  [unwired: 1 in, 2 out]
        "NIST Time" <- w487
        n216 = local read "Fast Data On"() -> (w478:bool)
        n217 = Not(x=w475) -> (.not. x?=w477:bool)
        n218 = Equal?(x=w485, y=w487) -> (x = y?=w486:bool)
        "NIST Time Failed to Read" <- w486
        n219 = And(x=w478, y=w477) -> (x .and. y?=w476:bool)
        n220 = Select(t=w485, s=w486, f=w487) -> (s? t:f=w488:u64)
        n221 = case shown="True" w476 {
          tunnel: w474 -> [_ w489]
          frame False {
          }
          frame True {
            n222 = To Double Precision Float(number=w489) -> (double precision float=w490:dbl)
            n223 = Multiply(x=2e-08, y=w490) -> (x*y=w492:dbl)
            n224 = To Unsigned Quad Integer(1:w492) -> (0:→"FPGA Timestamp (s)":u64)
          }
        }
        n225 = local read "Write Enable"() -> (w483:bool)
        n226 = Select(t=enum16{"Wait", "Get NIST Time", "Write"}."Write", s=w483, f=enum16{"Wait", "Get NIST Time", "Write"}."Wait") -> (s? t:f=w480:enum16{"Wait", "Get NIST Time", "Write"})
      }
      frame "Write" {
        n227 = local read "Fast Data On"() -> (w495:bool)
        n228 = local read "Slow Control On"() -> (w494:bool)
        n229 = Format Into String(initial string="NIST Time: ", w498) -> (resulting string=w500:string)  [unwired: 2 in, 1 out]
        n230 = case shown="True" w495 {
          tunnel: w498 -> [_ w512]
          tunnel: ["" w510] -> w499
          frame False {
          }
          frame True {
            n231 = local read "FPGA Timestamp (s)"() -> (w513:u64)
            n232 = Subtract(x=w512, y=w513) -> (x-y=w511:u64)
            n233 = Format Into String(initial string="FPGA Time: ", w513) -> (resulting string=w514:string)  [unwired: 2 in, 1 out]
            n234 = Format Into String(initial string="FPGA Drift: ", w511) -> (resulting string=w507:string)  [unwired: 2 in, 1 out]
            n235 = Concatenate Strings(w514, w507) -> (w510:string)
          }
        }
        n236 = case shown="True" w494 {
          tunnel: w498 -> [_ w520]
          tunnel: ["" w516] -> w497
          frame False {
          }
          frame True {
            n237 = local read "Slow time"() -> (w523:u64)
            n238 = Subtract(x=w520, y=w523) -> (x-y=w519:u64)
            n239 = Format Into String(initial string="Slow Drift: ", w519) -> (resulting string=w517:string)  [unwired: 2 in, 1 out]
            n240 = Format Into String(initial string="Slow Data Time: ", w523) -> (resulting string=w518:string)  [unwired: 2 in, 1 out]
            n241 = Concatenate Strings(w518, w517) -> (w516:string)
          }
        }
        n242 = Concatenate Strings(w500, w499, w497, "\r\n") -> (w502:string)
        n243 = Write to Text File(file (use dialog)=w504, text=w502) -> (refnum out=w503:refnum<file>)  [unwired: 2 in, 2 out]
      }
    }
  }
  n244 = case shown="True" w6 {
    tunnel: w13 -> [_ _]
    tunnel: [_ w525] -> w4
    tunnel: w7 -> [_ w526]
    frame False {
    }
    frame True {
      n245 = local read "IP Address of NIST Time Server"() -> (w528:string)
      n246 = call "XML_fast.vi"("Channel Cluster"="Channel Cluster", "DAQ Info Cluster"="DAQ Info Cluster", "Testpulse Cluster"="Testpulse Cluster", "IP Address of NIST Time Server"=w528, "NIST Time"=w526, "General Cluster"="General Cluster") -> ("XML String"=w525:string)  [unwired: 5 in]
      "XML String" <- w525
    }
  }
  n247 = local read "Slow Control On"() -> (w5:bool)
  n248 = case shown="True" w5 {
    tunnel: w4 -> [_ w534]
    tunnel: [_ w535] -> w3
    frame False {
    }
    frame True {
      w536 = "\r\n"
      n249 = local read "Slow Cluster"() -> (w532:T6)
      n250 = call "XML_slow.vi"("Slow Cluster"=w532, "Input String"="") -> ("Output String"=w533:string)
      n251 = Concatenate Strings(w534, w536, w533, w536) -> (w535:string)
      "Slow XML" <- w535
    }
  }
  n252 = local read "Write Enable"() -> (w2:bool)
  n253 = case shown="True" w2 {
    tunnel: w12 -> [_ w543]
    tunnel: w3 -> [_ w540]
    tunnel: w1 -> [_ w537]
    frame False {
    }
    frame True {
      n254 = Concatenate Strings(w540, "</mod>" ("string")) -> (w538:string)
      n255 = call "UTF8 LV80.vi"("text"=w538) -> ("utf-8 text out"=w542:string)
      n256 = Write to Text File(file (use dialog)=w543, text=w542) -> (refnum out=w541:refnum<file>)  [unwired: 2 in, 2 out]
      n257 = Close File(refnum=w537) -> ()  [unwired: 1 in, 2 out]
      n258 = Close File(refnum=w541) -> ()  [unwired: 1 in, 2 out]
    }
  }
